vi "invoke method in parallel.vi"(4 "results reporter":refnum<class "results reporter.lvclass">, 5 "execution system":T1=enum."standard", 6 "task token":refnum<class "null task token.lvclass">, 7 "ID":string, 8 "error in":errorcluster, 9 "parameters":variant, 10 "VI in":refnum<vi>, 11 "reporter":refnum<data-value>) -> (0 "error out":errorcluster, 3 "dispatcher out":refnum<data-value>)   [LabVIEW 2013, in "call function by reference.lvclass"]
uses:
  call function by reference.lvclass
  task token/null task token.lvclass
  dispatcher/thread pool.lvclass
  dispatcher/execution system.ctl
  results reporter/results reporter.lvclass
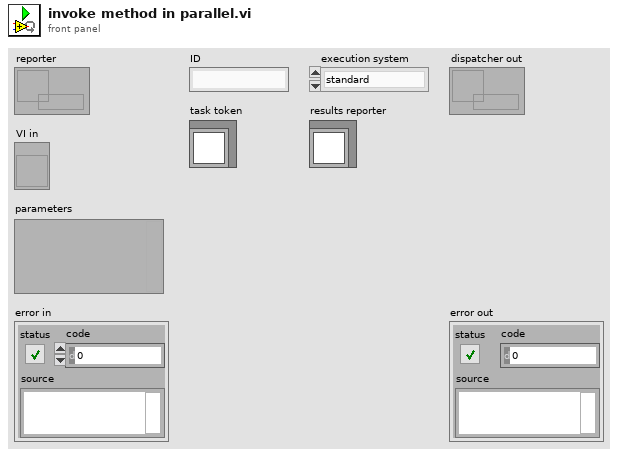
[diagram p1: front panel]
types:
  T1 = typedef "thread pool.lvclass/execution system.ctl" = enum32{"user interface", "standard", "instrument i/o", "data acquisition", "other 1", "other 2"}
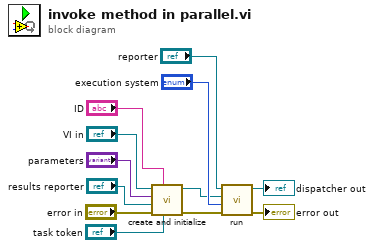
[diagram p0: block diagram]
diagram:
  n1 = call "create and initialize.vi"("task token"="task token", "task name"="ID", "error in"="error in", "results reporter"="results reporter", "parameters"="parameters", "function"="VI in") -> ("error out"=w12:errorcluster, "call by reference action"=w3:refnum<class "call function by reference.lvclass">)  [unwired: 4 in]
  n2 = call "run.vi"("error in"=w12, "execution system"="execution system", "task"=w3, "dispatcher"="reporter") -> ("error out"=→"error out":errorcluster, "dispatcher out"=→"dispatcher out":refnum<data-value>)  [unwired: 6 in]
